vi "日志报警状态存储 (子VI).vi"() -> ()   [LabVIEW 2016, in "斯坦道CODMn.lvlib"]
uses:
  <vilib>/ptbypt/NI_PtbyPt.lvlib
panel:
  out "多列列表框":i32(listbox)
  out "CODMn工作状态":T1(ring)
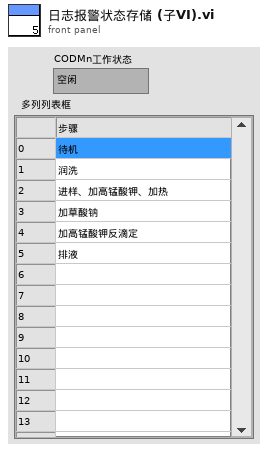
[diagram p1: front panel]
types:
  T1 = enum16{"空闲", "水样测试", "标样核查", "零点核查", "跨度核查", "空白测试", "平行样测试", "质控样", "空白校准", "标样校准", "加标回收"}
  T2 = cluster{"时间标识":timestamp, "参数":string, "日志信息":string, "流程参数":string}
  T3 = cluster{"ORP故障":bool, "温控器故障":bool, "加热故障":bool, "高锰酸钾报警":bool, "草酸钠报警":bool, "测量错误":bool, "校零错误":bool, "校标错误":bool, " 进水样超量程":bool, "排液阀故障":bool, "60分钟超时报警":bool, "进样无液体报警":bool}
  T4 = cluster{"测量量程":dbl, "测量精度":dbl, "测量间隔":dbl, "消解温度":dbl, "消解时长":dbl, "空白校准时间":timestamp, "曲线截距":dbl, "曲线斜率":dbl, "测量检出限":dbl, "测量信号值":dbl, "线性相关系数":dbl, "二次多项式系数":dbl, "标样校准时间":timestamp, "稀释倍数":dbl, "三项式系数":dbl, "空白标定系数":dbl, "量程系数":dbl, "F0/ORPA":dbl, "F1/ORPB":dbl, "F2/ORPK":dbl, "F3":dbl, "F4":dbl, "F5":dbl, "F6":dbl, "F7":dbl, "X0/滴定数":dbl, "量程":dbl}
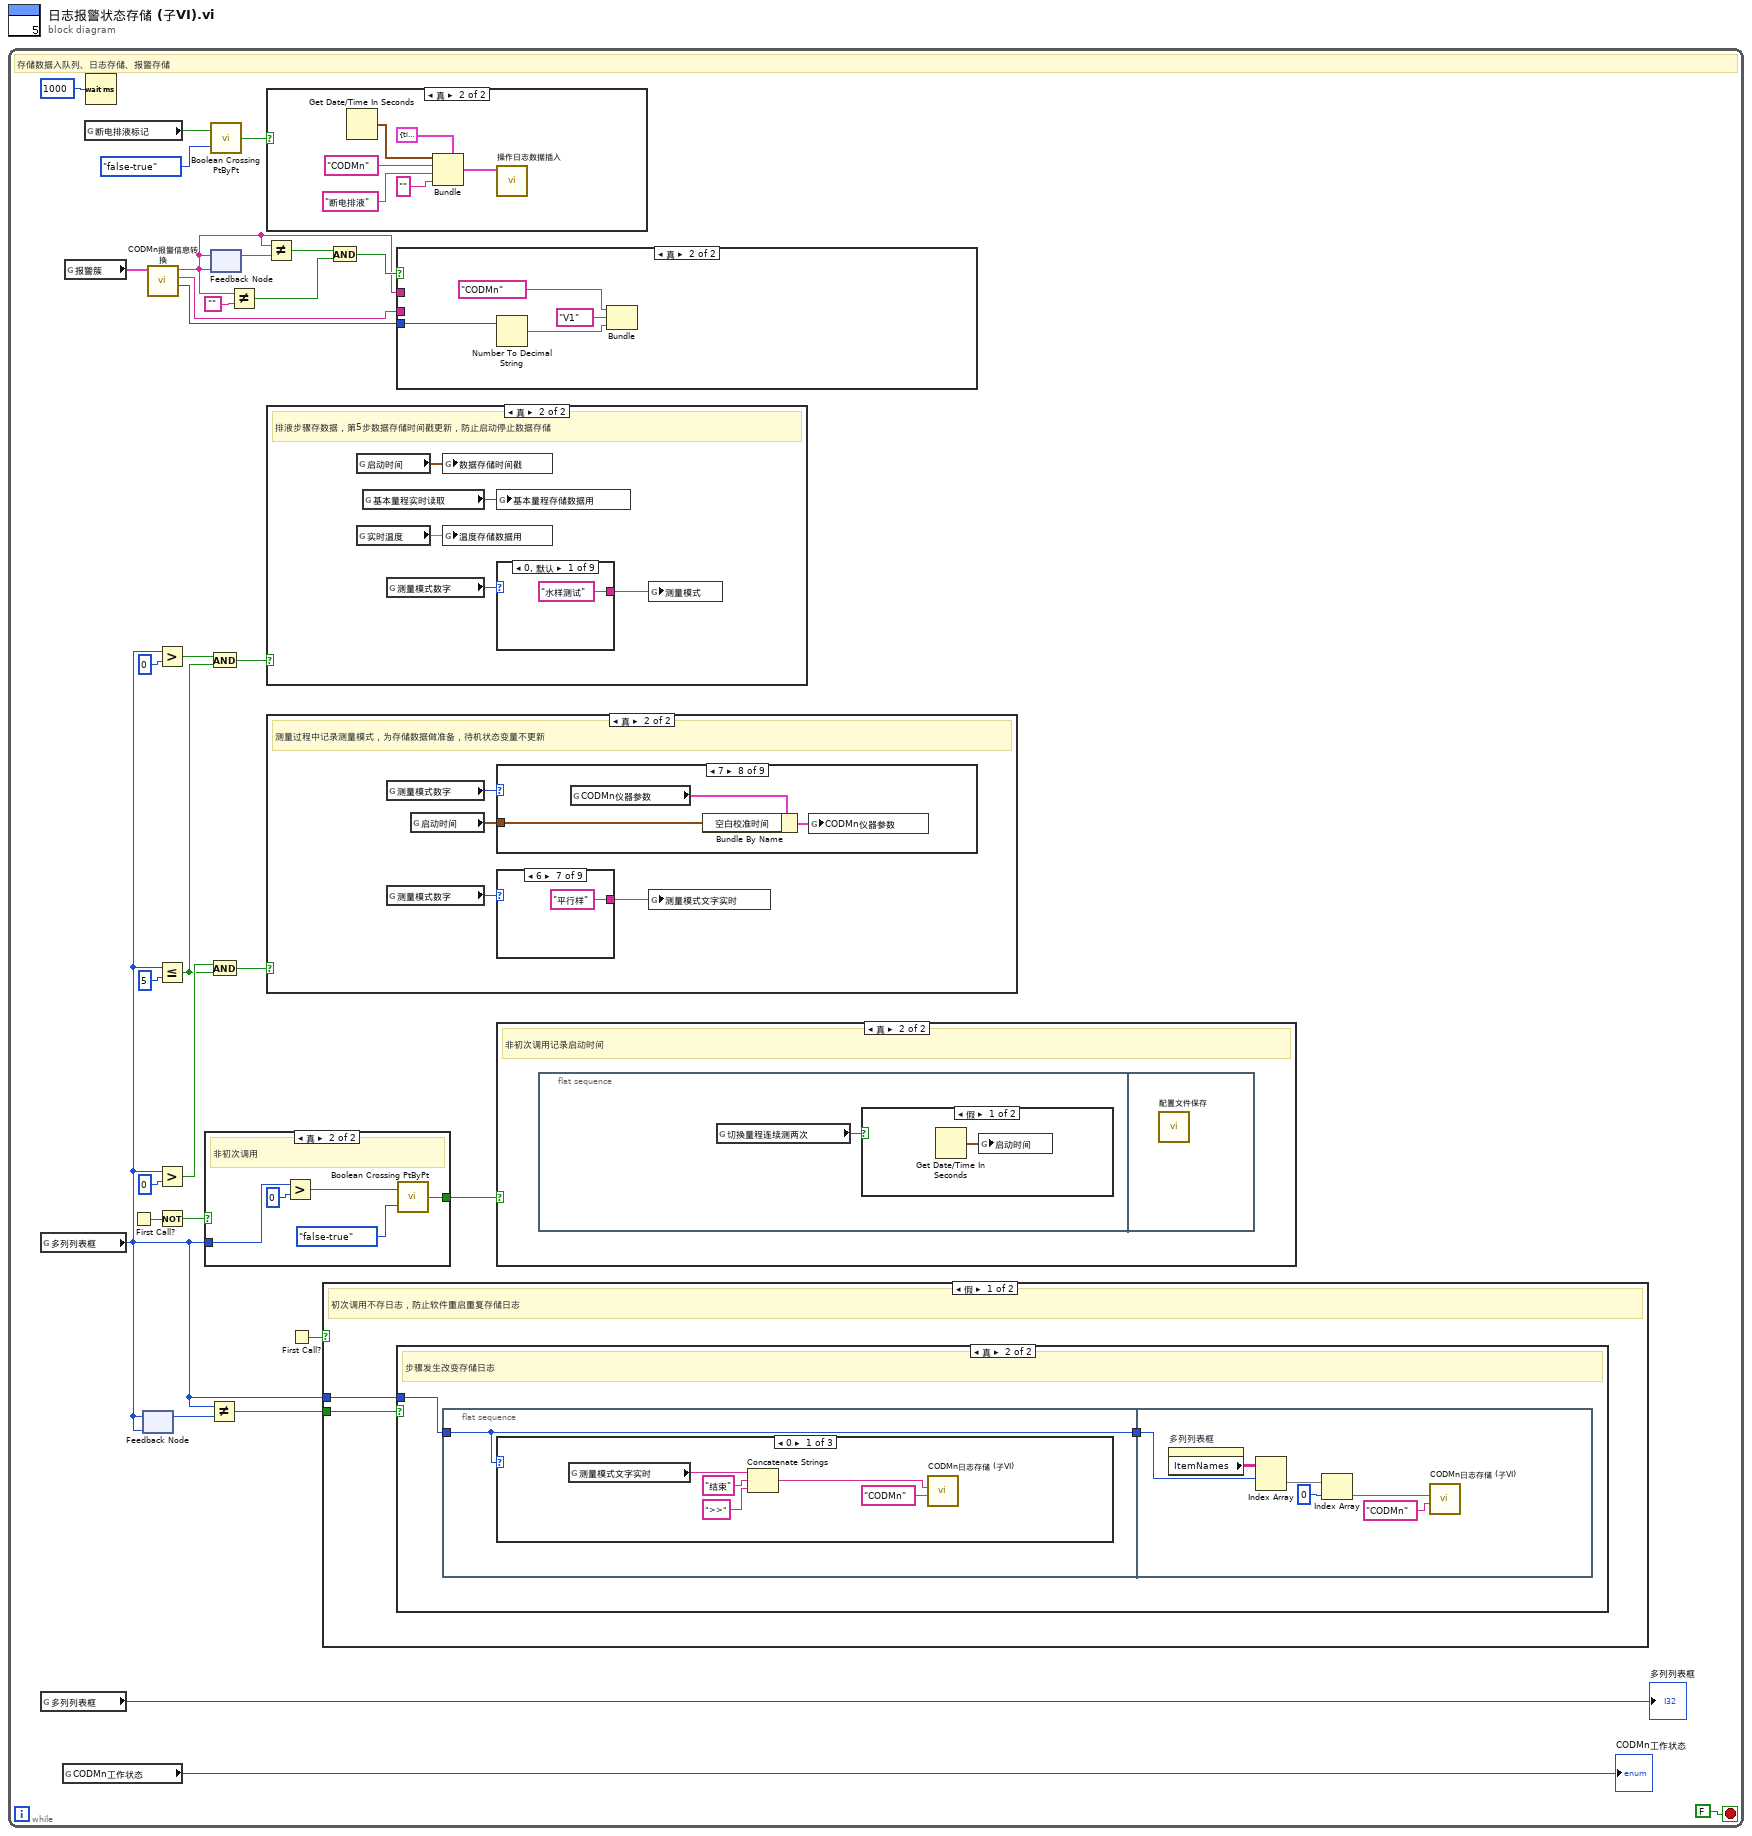
[diagram p0: block diagram]
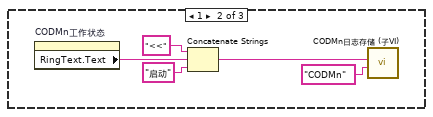
[diagram p3: hidden frame]
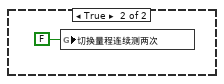
[diagram p10: hidden frame]
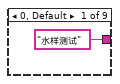
[diagram p12: hidden frame]
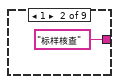
[diagram p13: hidden frame]
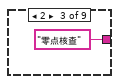
[diagram p14: hidden frame]
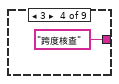
[diagram p15: hidden frame]
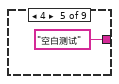
[diagram p16: hidden frame]
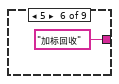
[diagram p17: hidden frame]
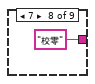
[diagram p18: hidden frame]
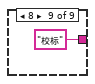
[diagram p19: hidden frame]
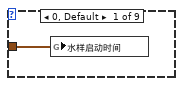
[diagram p20: hidden frame]
diagram:
  n1 = while {
    stop <- FALSE stop-if-true
    # "存储数据入队列、日志存储、报警存储"
    n2 = global read "运行时序全局变量.vi" "多列列表框"() -> (w5:i32)
    n3 = global read "运行时序全局变量.vi" "多列列表框"() -> (→"多列列表框":i32)
    n4 = global read "COD测量模式全局.vi" "CODMn工作状态"() -> (→"CODMn工作状态":T1)
    n5 = global read "COD内部交互全局.vi" "报警簇"() -> (w12:T3)
    n6 = global read "COD内部交互全局.vi" "断电排液标记"() -> (w11:bool)
    n7 = Wait (ms)(milliseconds to wait=u32 1000 ("等待时间（毫秒）")) -> ()  [unwired: 1 out]
    n8 = First Call?() -> (First Call?: T/F=w15:bool)
    n9 = feedback #1(w5) -> (w26:i32)
    n10 = feedback-in #1(w5) -> ()
    n11 = call "CODMn报警信息转换.vi"("报警簇"=w12) -> ("code"=w1:i32, "CODMN报警信息备注"=w2:string, "CODMN报警信息"=w16:string)  [unwired: 8 in]
    n12 = Greater?(x=w5, y=u16 0) -> (0:w7:bool)
    n13 = Less Or Equal?(x=w5, y=u16 5) -> (x <= y?=w6:bool)
    n14 = Greater?(x=w5, y=u16 0) -> (0:w31:bool)
    n15 = Not(x=w15) -> (.not. x?=w13:bool)
    n16 = case shown="真" w13 {
      selector: w13 -> [w53 _]
      tunnel: w5 -> [_ w55]
      tunnel: [w53 w54] -> w14
      frame False {
      }
      frame True {
        # "非初次调用"
        n17 = Greater?(x=w55, y=u16 0) -> (0:w58:bool)
        n18 = call <vilib>:"Boolean Crossing PtByPt.vi"("direction"=enum16{"either", "false-true", "true-false"}."false-true", "input"=w58) -> ("crossing"=w54:bool)  [unwired: 1 in]
      }
    }
    n19 = Not Equal?(x=w5, y=w26) -> (x != y?=w27:bool)
    n20 = And(x=w7, y=w6) -> (x .and. y?=w4:bool)
    n21 = And(x=w31, y=w6) -> (x .and. y?=w3:bool)
    n22 = call <vilib>:"Boolean Crossing PtByPt.vi"("direction"=enum16{"either", "false-true", "true-false"}."false-true", "input"=w11) -> ("crossing"=w22:bool)  [unwired: 1 in]
    n23 = feedback #2(w16) -> (w17:string)
    n24 = feedback-in #2(w16) -> ()
    n25 = Not Equal?(x=w16, y="") -> (x != y?=w21:bool)
    n26 = Not Equal?(x=w16, y=w17) -> (x != y?=w18:bool)
    n27 = case shown="真" w22 {
      frame False {
      }
      frame True {
        n28 = Get Date/Time In Seconds() -> (seconds since 1Jan1904=w68:timestamp)
        n29 = Bundle(cluster=T2 {"时间标识"=timestamp(0 s since 1904-01-01), "参数"="", "日志信息"="", "流程参数"=""} ("data in"), "时间标识"=w68, "参数"="CODMn" ("table输入"), "日志信息"="断电排液", "流程参数"="" ("table输入")) -> (w63:T2)
        n30 = call "操作日志数据插入.vi"("data"=w63) -> ()  [unwired: 9 in, 1 out]
      }
    }
    n31 = case shown="真" w4 {
      frame False {
      }
      frame True {
        # "排液步骤存数据，第5步数据存储时间戳更新，防止启动停止数据存储"
        n32 = global read "CODMn断电保存全局变量.vi" "启动时间"() -> (w97:timestamp)
        n33 = global read "COD内部交互全局.vi" "实时温度"() -> (w96:dbl)
        n34 = global read "COD内部交互全局.vi" "基本量程实时读取"() -> (w95:enum16{"L", "H", "AUTO"})
        n35 = global read "COD内部交互全局.vi" "测量模式数字"() -> (w94:i32)
        n36 = global write "COD内部交互全局.vi" "数据存储时间戳"(w97) -> ()
        n37 = global write "COD内部交互全局.vi" "温度存储数据用"(w96) -> ()
        n38 = global write "COD内部交互全局.vi" "基本量程存储数据用"(w95) -> ()
        n39 = case shown="0, 默认" w94 {
          tunnel: ["水样测试" ("测量模式") "标样核查" ("测量模式") "零点核查" ("测量模式") "跨度核查" ("测量模式") "空白测试" ("测量模式") "加标回收" ("测量模式") "平行样" ("测量模式") "校零" ("测量模式") "校标" ("测量模式")] -> w93
          frame 0, Default {
          }
          frame 1 {
          }
          frame 2 {
          }
          frame 3 {
          }
          frame 4 {
          }
          frame 5 {
          }
          frame 6 {
          }
          frame 7 {
          }
          frame 8 {
          }
        }
        n40 = global write "CODMn断电保存全局变量.vi" "测量模式"(w93) -> ()
      }
    }
    n41 = case shown="真" w3 {
      frame False {
      }
      frame True {
        # "测量过程中记录测量模式，为存储数据做准备，待机状态变量不更新"
        n42 = global read "COD内部交互全局.vi" "测量模式数字"() -> (w74:i32)
        n43 = global read "COD内部交互全局.vi" "测量模式数字"() -> (w72:i32)
        n44 = global read "CODMn断电保存全局变量.vi" "启动时间"() -> (w75:timestamp)
        n45 = case shown="7" w74 {
          tunnel: w75 -> [w85 _ _ _ _ w86 _ w87 w90]
          frame 0, Default {
            n46 = global write "COD测量模式全局.vi" "水样启动时间"(w85) -> ()
          }
          frame 1 {
          }
          frame 2 {
          }
          frame 3 {
          }
          frame 4 {
          }
          frame 5 {
            n47 = global write "COD测量模式全局.vi" "加标回收启动时间"(w86) -> ()
          }
          frame 6 {
          }
          frame 7 {
            n48 = global read "CODMn断电保存全局变量.vi" "CODMn仪器参数"() -> (w89:T4)
            n49 = Bundle By Name(cluster=w89, "空白校准时间"=w87) -> (w88:T4)
            n50 = global write "CODMn断电保存全局变量.vi" "CODMn仪器参数"(w88) -> ()
          }
          frame 8 {
            n51 = global read "CODMn断电保存全局变量.vi" "CODMn仪器参数"() -> (w92:T4)
            n52 = Bundle By Name(cluster=w92, "标样校准时间"=w90) -> (w91:T4)
            n53 = global write "CODMn断电保存全局变量.vi" "CODMn仪器参数"(w91) -> ()
          }
        }
        n54 = case shown="6" w72 {
          tunnel: ["水样测试" ("测量模式") "标样核查" ("测量模式") "零点核查" ("测量模式") "跨度核查" ("测量模式") "空白测试" ("测量模式") "加标回收" ("测量模式") "平行样" ("测量模式") "校零" ("测量模式") "校标" ("测量模式")] -> w73
          frame 0, Default {
          }
          frame 1 {
          }
          frame 2 {
          }
          frame 3 {
          }
          frame 4 {
          }
          frame 5 {
          }
          frame 6 {
          }
          frame 7 {
          }
          frame 8 {
          }
        }
        n55 = global write "COD测量模式全局.vi" "测量模式文字实时"(w73) -> ()
      }
    }
    n56 = First Call?() -> (First Call?: T/F=w28:bool)
    n57 = case shown="假" w28 {
      tunnel: w27 -> [w33 _]
      tunnel: w5 -> [w32 _]
      frame False {
        # "初次调用不存日志，防止软件重启重复存储日志"
        n58 = case shown="真" w33 {
          tunnel: w32 -> [_ w35]
          frame False {
          }
          frame True {
            # "步骤发生改变存储日志"
            n59 = flat-sequence {
              tunnel: w35 -> [w36]
              tunnel: [w36] -> w34
              tunnel: w34 -> [w52]
              frame #0 {
                n60 = case shown="0" w36 {
                  frame 0 {
                    n61 = global read "COD测量模式全局.vi" "测量模式文字实时"() -> (w38:string)
                    n62 = Concatenate Strings(w38, "结束" ("字符串"), ">>") -> (w41:string)
                    n63 = call "CODMn日志存储 (子VI).vi"("参数"="CODMn" ("table输入"), "日志信息"=w41) -> ()  [unwired: 10 in]
                  }
                  frame 1 {
                    n64 = property on="CODMn工作状态" class="Enum (严格)"() -> ("RingText.Text"=w42:string)  [unwired: 2 in, 2 out]
                    n65 = Concatenate Strings("<<", w42, "启动" ("字符串")) -> (w43:string)
                    n66 = call "CODMn日志存储 (子VI).vi"("参数"="CODMn" ("table输入"), "日志信息"=w43) -> ()  [unwired: 10 in]
                  }
                  frame 2, Default {
                  }
                }
              }
              frame #1 {
                n67 = property on="多列列表框" class="MCListbox (严格)"() -> ("ItemNames"=w47:string[][])  [unwired: 2 in, 2 out]
                n68 = Index Array(array=w47, index (row)=w52) -> (element=w50:string[])  [unwired: 1 in]
                n69 = Index Array(array=w50, index=0 ("索引")) -> (element=w48:string)
                n70 = call "CODMn日志存储 (子VI).vi"("参数"="CODMn" ("table输入"), "日志信息"=w48) -> ()  [unwired: 10 in]
              }
            }
          }
        }
      }
      frame True {
      }
    }
    n71 = And(x=w18, y=w21) -> (x .and. y?=w19:bool)
    n72 = case shown="真" w19 {
      tunnel: w16 -> [_ _]
      tunnel: w2 -> [_ _]
      tunnel: w1 -> [_ w62]
      frame False {
      }
      frame True {
        n73 = Number To Decimal String(number=w62) -> (decimal integer string=w59:string)  [unwired: 1 in]
        n74 = Bundle("componentParent"="CODMn", "equipVersion"="V1", w59) -> ()  [unwired: 1 in, 1 out]
      }
    }
    n75 = case shown="真" w14 {
      frame False {
      }
      frame True {
        # "非初次调用记录启动时间"
        n76 = flat-sequence {
          frame #0 {
            n77 = global read "COD内部交互全局.vi" "切换量程连续测两次"() -> (w69:bool)
            n78 = case shown="假" w69 {
              frame False {
                n79 = Get Date/Time In Seconds() -> (seconds since 1Jan1904=w70:timestamp)
                n80 = global write "CODMn断电保存全局变量.vi" "启动时间"(w70) -> ()
              }
              frame True {
                n81 = global write "COD内部交互全局.vi" "切换量程连续测两次"(FALSE ("切换量程连续测两次")) -> ()
              }
            }
          }
          frame #1 {
            n82 = call "配置文件保存.vi"() -> ()  [unwired: 12 in]
          }
        }
      }
    }
  }
